vi "ArduinoSerialRead.vi"() -> ()   [LabVIEW 2010]
uses:
  <vilib>/Utility/error.llb/DialogType.ctl
  <vilib>/_DAQmxBase/Internals/DAQmxBase Create Channel (AI-Voltage-Basic).vi
  <vilib>/_DAQmxBase/Internals/DAQmxBase Read (Analog 1D DBL NChan 1Samp).vi
panel:
  out "Waveform Graph":dbl[](graph)
  out "element":dbl
  in  "Port":tag="Dev1/port0"
  in  "stop":bool
  in  "Line":u8
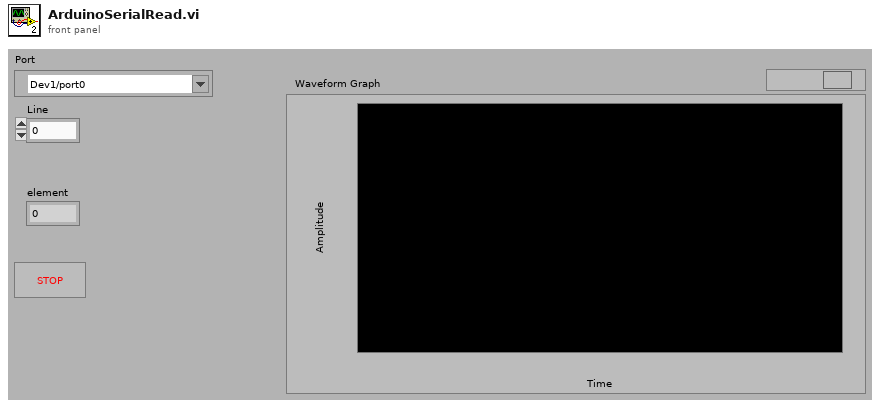
[diagram p1: front panel]
types:
  T1 = typedef "DialogType.ctl" = u16
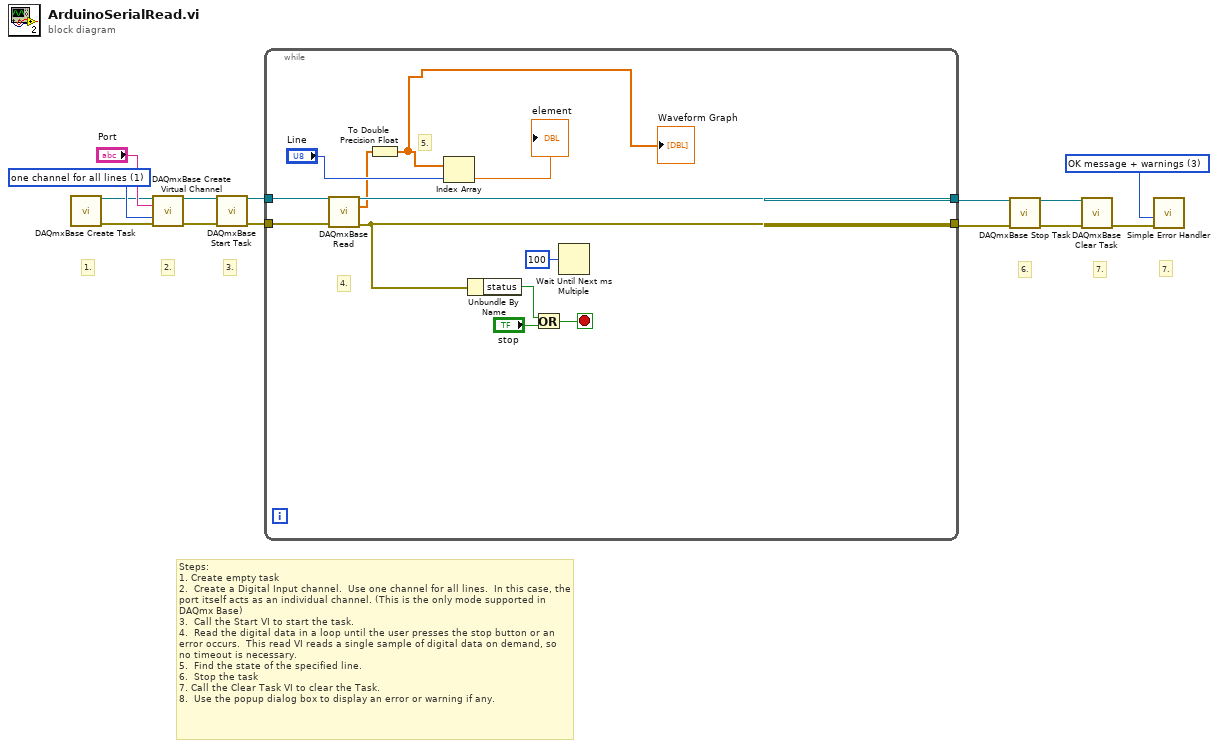
[diagram p0: block diagram]
diagram:
  w7 = 1 items=["one channel for each line", "one channel for all lines"] ("line grouping")
  w8 = T1 3 items=["no dialog", "OK message", "continue or stop message", "OK message + warnings", "continue/stop + warnings"] ("type of dialog (OK msg:1)")
  # "7."
  # "3."
  # "7."
  # "Steps: \n1. Create empty task\n2.  Create a Digital Input channel.  Use one channel for all lines.  In this case, the port itself acts as an individual channel. (This is the only mode supported in DAQmx Base)\n3.  Call the Start VI to start the task.\n4.  Read the digital data in a loop until the user presses the stop button or an error occurs.  This read VI reads a single sample of digital data on demand, so no timeout is necessary.\n5.  Find the state of the specified line.\n6.  Stop the task\n7. Call the Clear Task VI to clear the Task.\n8.  Use the popup dialog box to display an error or warning if any."
  # "6."
  # "2."
  # "1."
  n1 = call <vilib>:"DAQmxBase Create Task.vi"() -> ("task out"=w5:refnum<k21>, "error out"=w6:errorcluster)  [unwired: 14 in]
  n2 = call-poly <vilib>:"DAQmxBase Create Virtual Channel.vi"("task in"=w5, "physical channels"="Port", "units"=w7, "error in"=w6) -> ("task out"=w11:refnum<k21>, "error out"=w10:errorcluster)  [unwired: 10 in]
  n3 = call <vilib>:"DAQmxBase Start Task.vi"("task/channels in"=w11, "error in"=w10) -> ("task out"=w12:refnum<k21>, "error out"=w14:errorcluster)  [unwired: 12 in]
  n4 = while {
    tunnel: w14 -> [w26]
    tunnel: [w22] -> w4
    tunnel: w12 -> [w21]
    tunnel: [w20] -> w3
    stop <- w25 stop-if-true
    # "5."
    # "4."
    n5 = call-poly <vilib>:"DAQmxBase Read.vi"("task/channels in"=w21, "error in"=w26) -> ("task out"=w20:refnum<k21>, "data"=w17:dbl[], "error out"=w22:errorcluster)  [unwired: 11 in]
    n6 = To Double Precision Float(number=w17) -> (double precision float=w15:dbl[])
    "Waveform Graph" <- w15
    n7 = Index Array "Index Array"(array=w15, index="Line") -> (element=→"element":dbl)
    n8 = Unbundle By Name(w22) -> ("status"=w23:bool)
    n9 = Or(x=w23, y="stop") -> (x .or. y?=w25:bool)
    n10 = Wait Until Next ms Multiple(millisecond multiple=u32 100 ("milliseconds to wait")) -> ()  [unwired: 1 out]
  }
  n11 = call <vilib>:"DAQmxBase Stop Task.vi"("task/channels in"=w3, "error in"=w4) -> ("task out"=w2:refnum<k21>, "error out"=w1:errorcluster)  [unwired: 12 in]
  n12 = call <vilib>:"DAQmxBase Clear Task.vi"("task in"=w2, "error in"=w1) -> ("error out"=w13:errorcluster)  [unwired: 13 in]
  n13 = call <vilib>:"Simple Error Handler.vi"("type of dialog (OK msg:1)"=w8, "error in (no error)"=w13) -> ()  [unwired: 3 in, 5 out]
